vi "Set Range.vi"(6 "Range Cluster":T1, 8 "error in (no error)":errorcluster, 9 "Multiplot Representation In":T2, 10 "Actual Transform In":T6, 11 "3D Plot.lvclass in":refnum<class "3D Plot.lvclass">) -> (0 "error out":errorcluster, 1 "Multiplot Representation In":T2, 2 "Actual Transform Out":T6, 3 "3D Plot.lvclass out":refnum<class "3D Plot.lvclass">)   [LabVIEW 2020, in "3D Plot.lvclass"]
uses:
  <vilib>/Math Plots/3D Math Plots/3D Plot/3D Plot/3D Plot.lvclass
  <vilib>/Math Plots/3D Math Plots/3D Plot/3D Plot/Typedef/Actual Transform.ctl
  <vilib>/Math Plots/3D Math Plots/3D Plot/3D Plot/Typedef/Range Clusters.ctl
  <vilib>/Math Plots/3D Math Plots/3D Plot/3D Plot/Typedef/Multiplot Representation.ctl
  <vilib>/Math Plots/3D Math Plots/3D Plot/3D Plot/Typedef/Plot Representation.ctl
  <vilib>/Math Plots/3D Math Plots/3D Plot/3D Plot/Typedef/Mesh Data.ctl
  <vilib>/Math Plots/3D Math Plots/3D Plot/3D Plot/3D Plot.lvclass/3D Plot.ctl
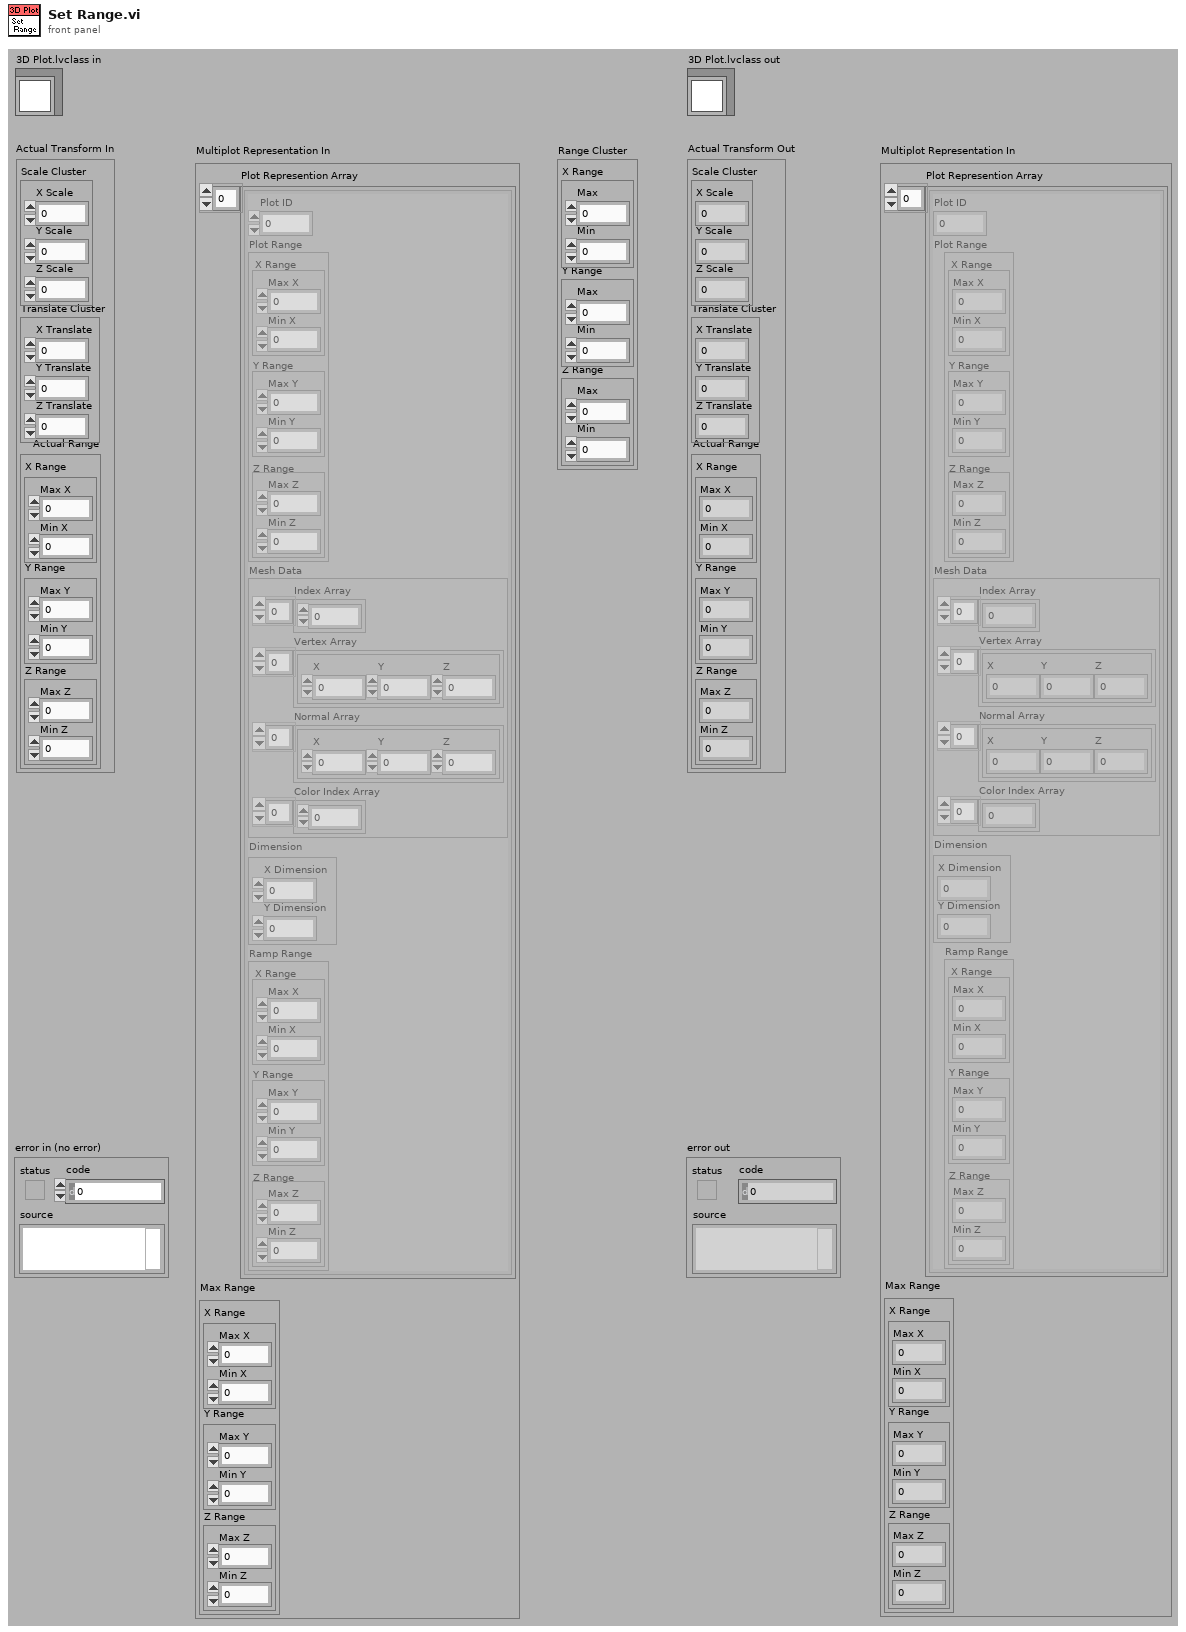
[diagram p1: front panel]
types:
  T1 = cluster{"X Range":cluster{"Max":sgl, "Min":sgl}, "Y Range":cluster{"Max":sgl, "Min":sgl}, "Z Range":cluster{"Max":sgl, "Min":sgl}}
  T2 = typedef "3D Plot.lvclass/Multiplot Representation.ctl" = cluster{"Plot Represention Array":T3[], "Max Range":T4}
  T3 = typedef "3D Plot.lvclass/Plot Representation.ctl" = cluster{"Plot ID":i32, "Plot Range":T4, "Mesh Data":T5, "Dimension":cluster{"X Dimension":i32, "Y Dimension":i32}, "Ramp Range":T4}
  T4 = typedef "3D Plot.lvclass/Range Clusters.ctl" = cluster{"X Range":cluster{"Max X":sgl, "Min X":sgl}, "Y Range":cluster{"Max Y":sgl, "Min Y":sgl}, "Z Range":cluster{"Max Z":sgl, "Min Z":sgl}}
  T5 = typedef "3D Plot.lvclass/Mesh Data.ctl" = cluster{"Index Array":u32[], "Vertex Array":cluster{"X":sgl, "Y":sgl, "Z":sgl}[], "Normal Array":cluster{"X":sgl, "Y":sgl, "Z":sgl}[], "Color Index Array":i32[]}
  T6 = typedef "3D Plot.lvclass/Actual Transform.ctl" = cluster{"Scale Cluster":cluster{"X Scale":sgl, "Y Scale":sgl, "Z Scale":sgl}, "Translate Cluster":cluster{"X Translate":sgl, "Y Translate":sgl, "Z Translate":sgl}, "Actual Range":T4}
  T7 = cluster{"Scale Out":sgl, "Scale Out":sgl, "Scale Out":sgl}
  T8 = cluster{"Translate Out":sgl, "Translate Out":sgl, "Translate Out":sgl}
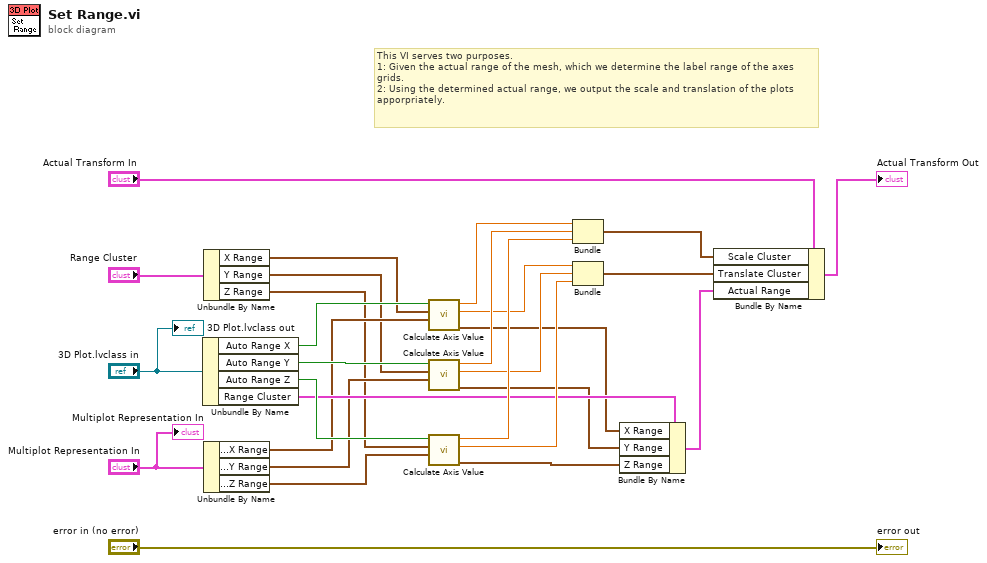
[diagram p0: block diagram]
diagram:
  # "This VI serves two purposes.  \n1: Given the actual range of the mesh, which we determine the label range of the axes grids.   \n2: Using the determined actual range, we output the scale and translation of the plots apporpriately."
  n1 = Unbundle By Name("3D Plot.lvclass in") -> ("Auto Range X"=w21:bool, "Auto Range Y"=w20:bool, "Auto Range Z"=w19:bool, "Range Cluster"=w11:T4)
  n2 = Unbundle By Name("Range Cluster") -> ("X Range"=w6:cluster{"Max":sgl, "Min":sgl}, "Y Range"=w5:cluster{"Max":sgl, "Min":sgl}, "Z Range"=w4:cluster{"Max":sgl, "Min":sgl})
  n3 = Unbundle By Name("Multiplot Representation In") -> ("Max Range.X Range"=w9:cluster{"Max X":sgl, "Min X":sgl}, "Max Range.Y Range"=w8:cluster{"Max Y":sgl, "Min Y":sgl}, "Max Range.Z Range"=w7:cluster{"Max Z":sgl, "Min Z":sgl})
  n4 = call <vilib>:"Calculate Axis Value.vi"("Plot Range"=w9, "Set Range"=w6, "Auto Range?"=w21) -> ("Actual Range Out"=w3:cluster{"Max":sgl, "Min":sgl}, "Translate Out"=w13:sgl, "Scale Out"=w14:sgl)  [unwired: 6 out]
  n5 = call <vilib>:"Calculate Axis Value.vi"("Plot Range"=w8, "Set Range"=w5, "Auto Range?"=w20) -> ("Actual Range Out"=w2:cluster{"Max":sgl, "Min":sgl}, "Translate Out"=w16:sgl, "Scale Out"=w15:sgl)  [unwired: 6 out]
  n6 = call <vilib>:"Calculate Axis Value.vi"("Plot Range"=w7, "Set Range"=w4, "Auto Range?"=w19) -> ("Actual Range Out"=w1:cluster{"Max":sgl, "Min":sgl}, "Translate Out"=w17:sgl, "Scale Out"=w18:sgl)  [unwired: 6 out]
  n7 = Bundle("Scale Out"=w14, "Scale Out"=w15, "Scale Out"=w18) -> (w22:T7)  [unwired: 1 out]
  n8 = Bundle("Translate Out"=w13, "Translate Out"=w16, "Translate Out"=w17) -> (w12:T8)  [unwired: 1 out]
  n9 = Bundle By Name(cluster=w11, "X Range"=w3, "Y Range"=w2, "Z Range"=w1) -> (w10:T4)
  n10 = Bundle By Name(cluster="Actual Transform In", "Scale Cluster"=w22, "Translate Cluster"=w12, "Actual Range"=w10) -> (→"Actual Transform Out":T6)
  "error out" <- "error in (no error)"
  "Multiplot Representation In" <- "Multiplot Representation In"
  "3D Plot.lvclass out" <- "3D Plot.lvclass in"
